vi "gl_Windows Ctrl refs.vi"() -> ()   [LabVIEW 2020]
uses:
  Subpanel Windows/SubVIs/Typedefs/Live window-ctrl refs.ctl
  Typedefs/Channel Selector.ctl
  Typedefs/Image display ref.ctl
  Movement Correction/Typedefs/Reference plots window ctrl refs.ctl
  Windows/Ref select window/Typedefs/Ref select window ctrl refs.ctl
panel:
  out "Refresh live img UI":bool
  in  "Linked sliders":bool
  out "Sliders distance (right)":i16
  out "Sliders distance (left)":i16
  in  "Slider distance locked (right)":bool
  in  "Slider distance locked (left)":bool
  in  "Ref select window ctrl refs":T1
  in  "Ref plots window ctrl refs":T2
  in  "MovCor Ref window ctrl refs":T3
  in  "Live img window ctrl refs":T3
  # "This is set TRUE when a user or user profile has been switched."
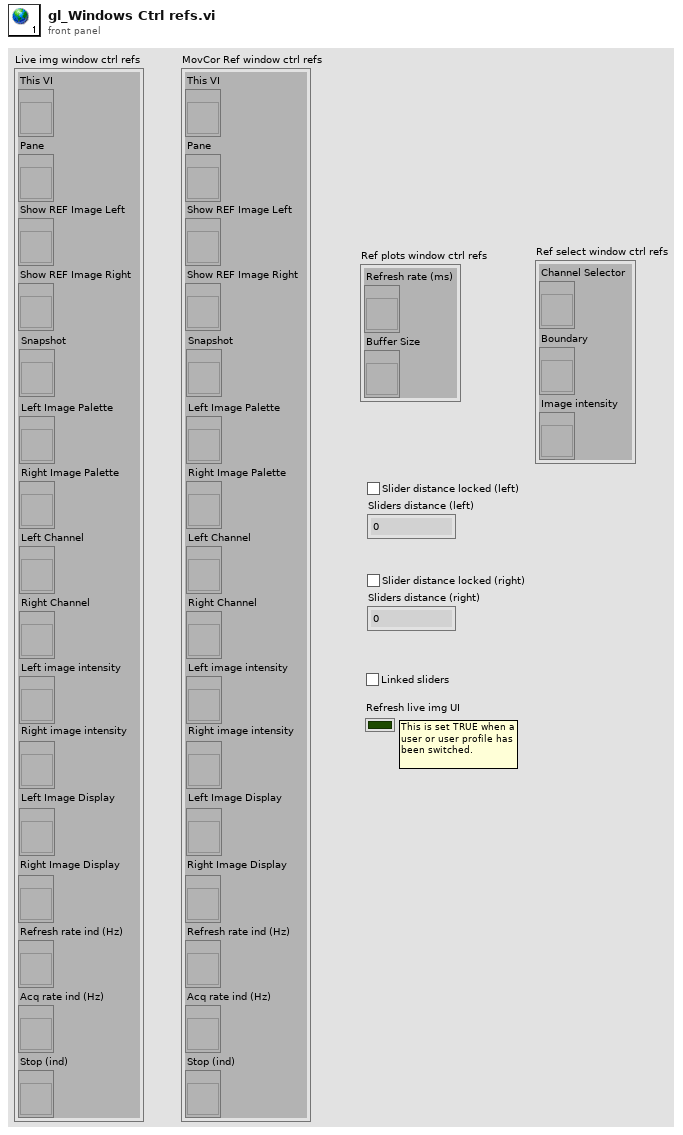
[diagram p1: front panel]
types:
  T1 = typedef "Ref select window ctrl refs.ctl" = cluster{"Channel Selector":refnum<vi>, "Boundary":refnum<vi>, "Image intensity":refnum<vi>}
  T2 = typedef "Reference plots window ctrl refs.ctl" = cluster{"Refresh rate (ms)":refnum<vi>, "Buffer Size":refnum<vi>}
  T3 = typedef "Live window-ctrl refs.ctl" = cluster{"This VI":refnum<vi>, "Pane":refnum<vi>, "Show REF Image Left":refnum<vi>, "Show REF Image Right":refnum<vi>, "Snapshot":refnum<vi>, "Left Image Palette":refnum<vi>, "Right Image Palette":refnum<vi>, "Left Channel":refnum<vi>, "Right Channel":refnum<vi>, "Left image intensity":refnum<vi>, "Right image intensity":refnum<vi>, "Left Image Display":T4, "Right Image Display":T4, "Refresh rate ind (Hz)":refnum<vi>, "Acq rate ind (Hz)":refnum<vi>, "Stop (ind)":refnum<vi>}
  T4 = typedef "Image display ref.ctl" = refnum<vi>
diagram:
